vi "deleteController_TCrane.vi"() -> ()   [LabVIEW 2009]
uses:
  <vilib>/Platform/TimedLoop/XDataNode/nitl_modes.ctl
  <vilib>/Utility/miscctls.llb/LVRGBAColorTypeDef.ctl
  Instance           2 23Saved   OpenLoop_TCrane .vi
  <vilib>/Instr/_visa.llb/VISA Configure Serial Port (Instr).vi
  <vilib>/Platform/TimedLoop/XDataNode/XDataNode.xnode
  <vilib>/Platform/TimedLoop/XDataNode/loadlvalarms.vi
  <vilib>/Platform/TimedLoop/XDataNode/timing_clust.ctl
  <vilib>/Platform/TimedLoop/XDataNode/wakeup.ctl
  Instance           3 23Saved   OpenLoop_TCrane .vi
  Instance           4 23Saved   OpenLoop_TCrane .vi
  Instance           5 23Saved   OpenLoop_TCrane .vi
  <vilib>/Utility/file.llb/Read From Spreadsheet File (string).vi
  <vilib>/Utility/file.llb/Write To Spreadsheet File (DBL).vi
  <vilib>/Utility/file.llb/Write To Spreadsheet File (string).vi
  <vilib>/Utility/miscctls.llb/LV3DPointTypeDef.ctl
  <vilib>/imath/engines/lvmath2/RunTimeEngine/ErrorHandling/NIMS_Finalize Error.vi
  <vilib>/imath/engines/lvmath2/RunTimeEngine/Parser/MC_Version.vi
  <vilib>/imath/engines/lvmath2/RunTimeEngine/NodeEndStatement/NIMS_NodeEndStatement_Output.vi
  <instcachedir>/1/NIMS_NodeEndStatement_Output_53EC0D466D134D7ABD903AC30B43404B.lvgen/NIMS_NodeEndStatement_Output_53EC0D466D134D7ABD903AC30B43404B_004.vi
  <vilib>/imath/engines/lvmath2/RunTimeEngine/BuiltInFunctions/abs/NIMS_abs(signed).vi
  <instcachedir>/1/NIMS_abs(signed)_C4FCB8E6058B49B797C7C8D53CA5F6EC.lvgen/NIMS_abs(signed)_C4FCB8E6058B49B797C7C8D53CA5F6EC_000.vi
  <vilib>/imath/engines/lvmath/Functions/Error Handling/MergeErrorsWrapper.vi
  <instcachedir>/1/NIMS_NodeEndStatement_Output_53EC0D466D134D7ABD903AC30B43404B.lvgen/NIMS_NodeEndStatement_Output_53EC0D466D134D7ABD903AC30B43404B_002.vi
  RTDACUSB_TCrane.dll
  <vilib>/Platform/TimedLoop/XDataNode/XDNodeRunTimeDep.lvlib
panel:
  in  "Tab Control":enum32{"Main", "I/O", "Advanced", "Wireless"}(tab)
  in  "Motors on":bool caption="Motors"
  in  "Camera Control 2":dbl(slide)=60.0 min=1.0 max=90.0 scale=90.0..1.0
  out "X displacement chart":dbl(graph)
  out "Y displacement chart":dbl(graph)
  out "Z displacement chart":dbl(graph)
  out "XY Graph":cluster{"Y":dbl[], "Y":dbl[]}[](graph)
  out "Alpha":dbl
  out "Beta":dbl
  out "3D view":refnum<vi>(3d-picture)
  in  "Camera Control":dbl(slide) scale=-180.0..180.0
  in  "Animation":bool
  in  "Controller:":u16(ring) items=["None", "P (Tracking)", "P (Delay Controller)", "PI (Tracking)", "PID (DelayController)"]
  in  "X":dbl
  in  "Stop Controller":bool
  in  "T":dbl min=0.0 max=3.14 step=0.05
  in  "Z":dbl
  in  "Referense Slide X":dbl(slide) scale=0.0..50.0
  in  "Referense Slide T":dbl(slide) scale=0.0..3.14
  in  "Referense Slide Z":dbl(slide) scale=0.0..100.0
  in  "Cont Switch X":bool
  in  "Cont Switch T":bool
  in  "Cont Switch Z":bool
  in  "stop 2":bool
  in  "Home":bool
  in  "Reset angles":bool
  in  "Motors off":bool
  in  "Timed Sequence":bool
  in  "Stop TIV":bool
  in  "Saving":bool
  in  "Stop saving":bool
  in  "Start saving":bool
  in  "Path":path
  in  "Load TIV 2":path
  out "TIV Table":string[][](table)
  in  "Load TIV":bool
  out "TIV active":bool
  in  "Run TIV+SAVE":bool
  in  "Input type":bool
  out "Control Sequence":bool
  out "Reference Series\n(Trajectory)":bool
  out "Switch at":dbl
  out "X Scope":dynamicdata(graph)
  out "Theta Scope":dynamicdata(graph)
  out "Z Scope":dynamicdata(graph)
  out "Waveform Chart":i32(graph)
  out "Sample time [ms]":dbl format="%#.12g"
  out "Counter pulses":dbl format="%#.12g"
  out "Time":dbl
  in  "Timer active":bool
  out "Encoder X":dbl format="%#.12g"
  in  "X-axis control":dbl(slide) scale=-1.0..1.0
  in  "X-Motor On/Off":bool
  out "X - Motor On/Off":bool
  out "Numeric":dbl
  out "No of detected boards":dbl
  out "Logic version":dbl
  out "Last error":string
  in  "Theta-angle control":dbl(slide) scale=-1.0..1.0
  in  "T-Motor On/Off":bool
  out "Theta - Motor On/Off":bool
  out "Numeric 2":dbl
  in  "Z-axis control":dbl(slide) scale=-1.0..1.0
  in  "Z-Motor On/Off":bool
  out "Z - Motor On/Off":bool
  out "Numeric 3":dbl
  out "Encoder Theta":dbl format="%#.12g"
  out "Encoder Z":dbl format="%#.12g"
  out "Encoder Alfa":dbl format="%#.12g"
  out "Encoder Beta":dbl format="%#.12g"
  in  "Limit flags":T1(radio)=enum."Radio Selection 2"
  in  "Therm flags":T2(radio)=enum."Radio Selection 2"
  in  "Stop motors":bool
  out "X-axis therm flag":bool
  out "T-angle therm flag":bool
  out "Z-axis therm flag":bool
  out "X-axis limit flag":bool
  out "T-angle limit flag":bool
  out "Z-axis limit flag":bool
  in  "Reset encoders":bool
  out "RESET value":dbl format="%#.12g"
  in  "Soft limit flags":bool=TRUE
  in  "k 1":dbl=0.4 step=0.1
  in  "k 2":dbl=0.4 step=0.1
  in  "Mode":T3=enum."Discard missed periods, maintain original phase"
  in  "Wireless Active":bool
  in  "Baud Rate":i32(ring)=6 items=["2400"=2400, "4800"=4800, "9600"=9600, "19200"=19200, "38400"=38400, "57600"=57600, "115200"=115200]
  in  "VISA resource name":refnum<visa-resource-name>="COM1"
  out "Float1":sgl
  out "Float2":sgl
  out "Float3":sgl
  out "Float4":sgl
  out "Current Ref Z":dbl
  out "Current Ref X":dbl
  out "Current Ref T":dbl
  in  "Offset Beta":dbl
  in  "Offset Alpha":dbl
  out "TIV size":i32
  out "Index":i32
  # "Time"
  # "X"
  # "Theta"
  # "Z"
  # "Please specify the Input type when loading the input data chart"
  # "RT-DAC/USB status"
  # "Tower Crane motor control"
  # "Controller Parameters"
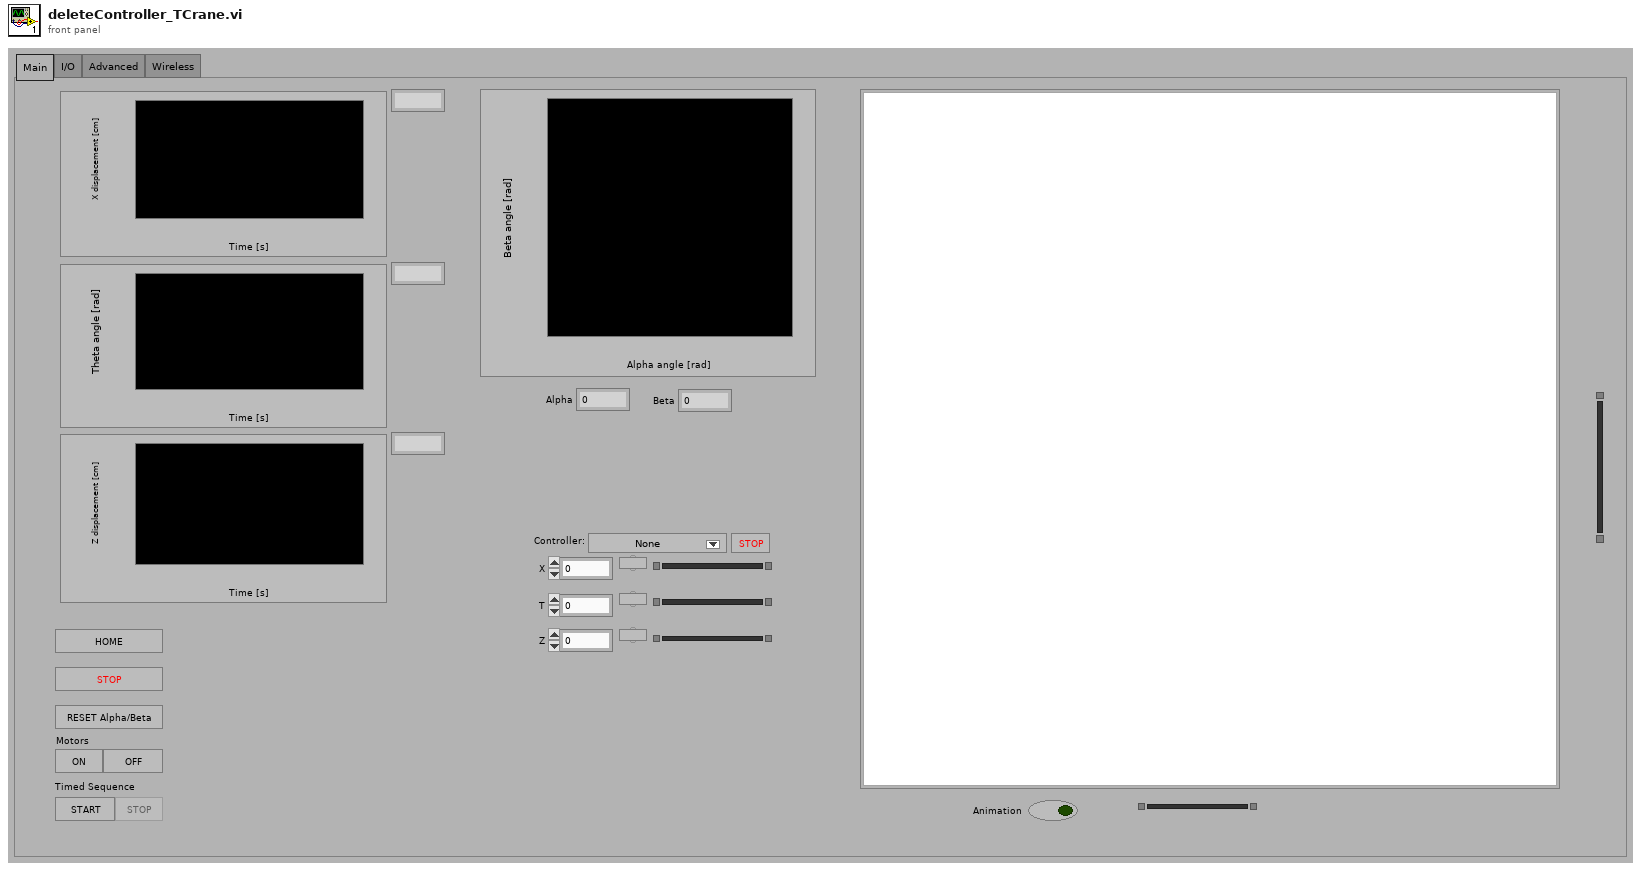
[diagram p1: front panel]
types:
  T1 = enum32{"Set limit flags to:", "Radio Selection 2"}
  T2 = enum32{"Set therm flags to:", "Radio Selection 2"}
  T3 = typedef "XDNodeRunTimeDep.lvlib/nitl_modes.ctl" = enum32{"No Change", "Process missed periods, maintain original phase", "Discard missed periods, maintain original phase", "Process missed periods, ignore original phase", "Discard missed periods, ignore original phase"}
  T4 = typedef "LVRGBAColorTypeDef.ctl" = cluster{"Red":sgl, "Green":sgl, "Blue":sgl, "Alpha":sgl}
  T5 = typedef "XDNodeRunTimeDep.lvlib/timing_clust.ctl" = cluster{"Expected End [f-1]":u64, "Actual End [f-1]":u64, "Finished Late? [f-1]":bool, "Expected End [i-1]":u64, "Actual End [i-1]":u64, "Finished Late? [i-1]":bool, "Expected Start [i]":u64, "Actual Start [i]":u64, "Expected Start [f]":u64, "Actual Start [f]":u64, "Source Name":string, "Structure Name":string, "Period":i64, "Deadline":i64, "Offset":i64, "Start":i64, "Priority":i32, "Timeout":i32, "Mode":T3, "Wakeup Reason":T6, "Error":errorcluster, "Source Type":string, "Secondary Source Type":string, "Global End Time":u64, "Global Start Time":u64, "Frame Duration":u64, "Iteration Duration":u64, "Assigned CPU":i32, "I/O Scan Engine Mode":u32}
  T6 = typedef "XDNodeRunTimeDep.lvlib/wakeup.ctl" = enum32{"Normal", "Aborted", "Asynchronous wakeup", "Timing source error", "Timed loop error", "Timeout"}
  T7 = typedef "LV3DPointTypeDef.ctl" = cluster{"X":sgl, "Y":sgl, "Z":sgl}
  T8 = enum8{"Enabled", "Disabled", "Disabled and Grayed Out"}
  T9 = cluster{"Numeric 2":dbl, "Numeric 3":dbl, "Numeric 4":dbl}
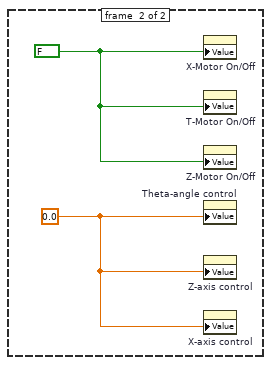
[diagram p2: hidden frame]
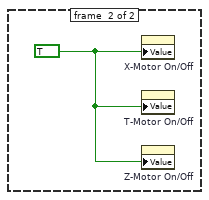
[diagram p3: hidden frame]
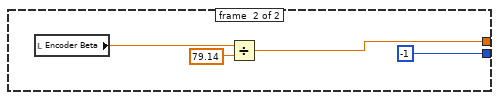
[diagram p4: hidden frame]
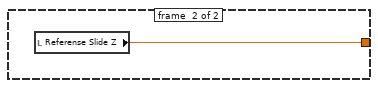
[diagram p5: hidden frame]
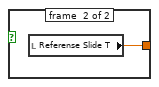
[diagram p6: hidden frame]
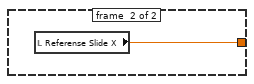
[diagram p7: hidden frame]
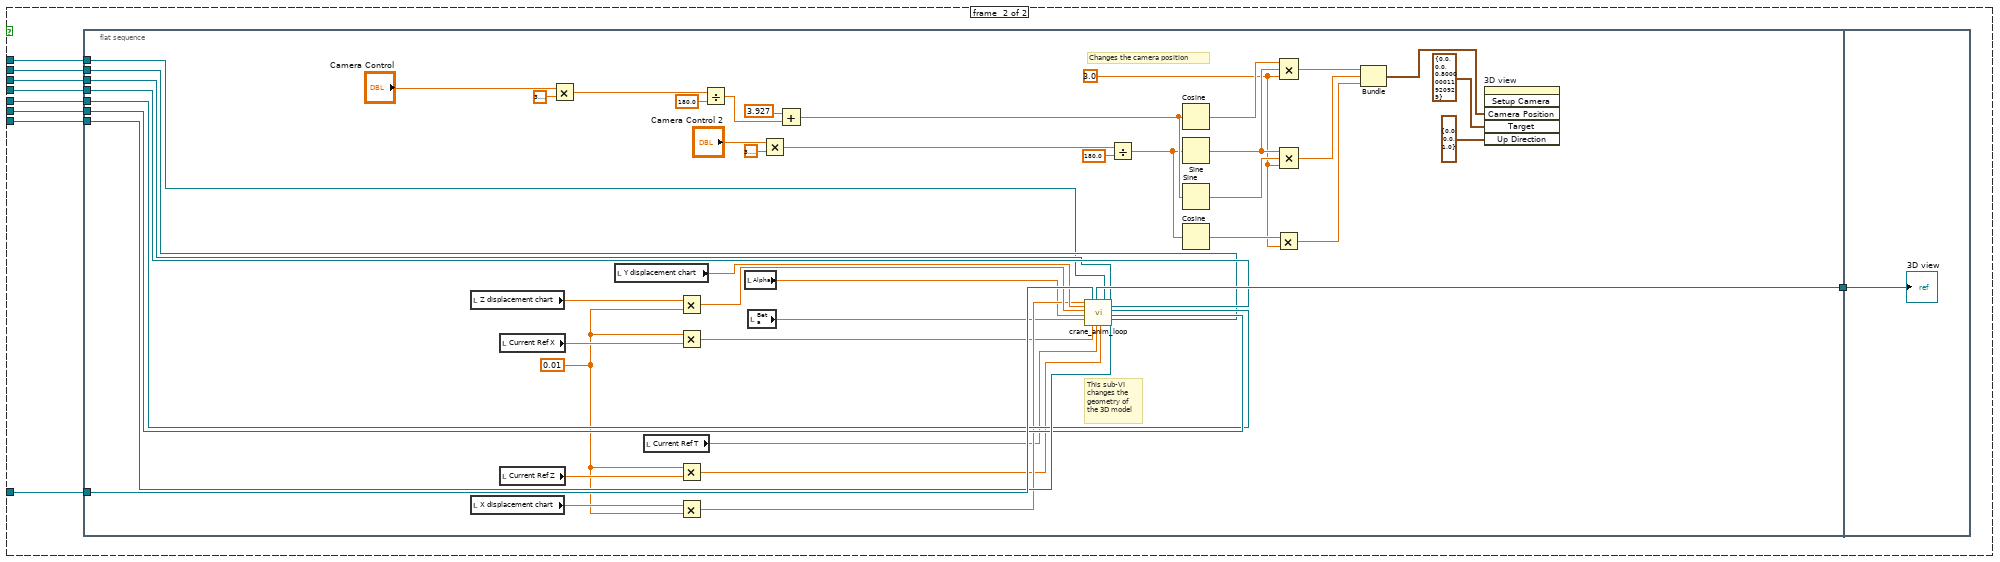
[diagram p8: hidden frame]
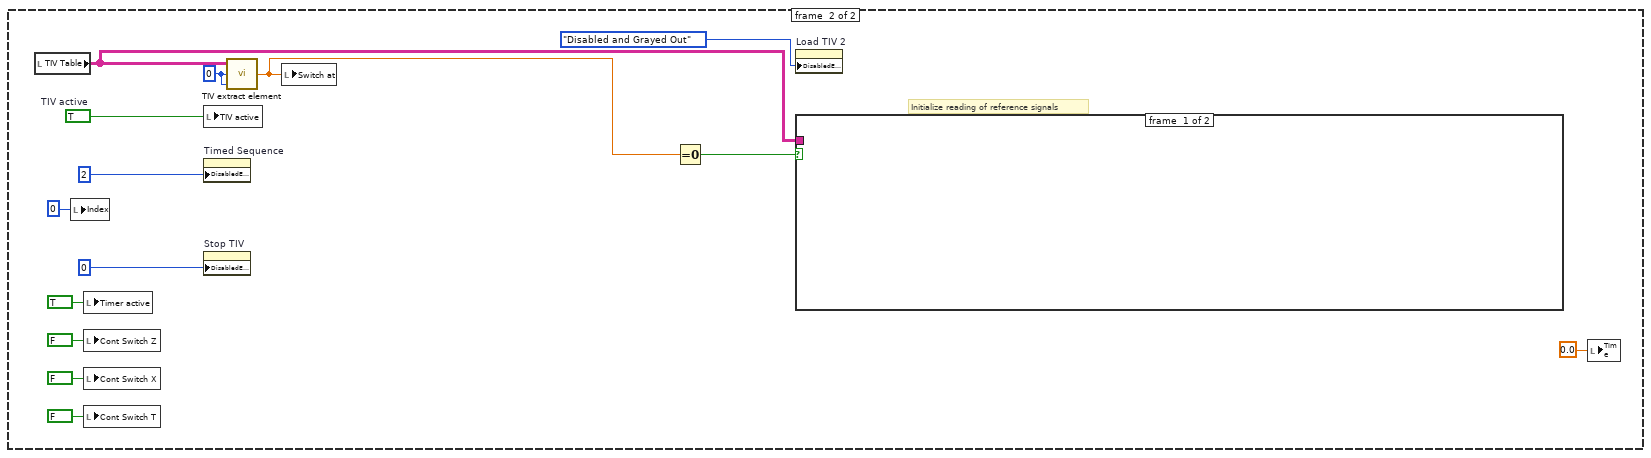
[diagram p9: hidden frame]
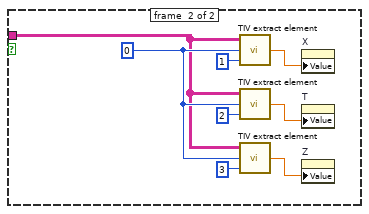
[diagram p10: hidden frame]
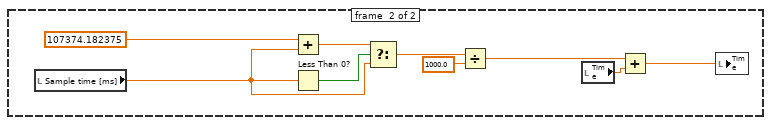
[diagram p11: hidden frame]
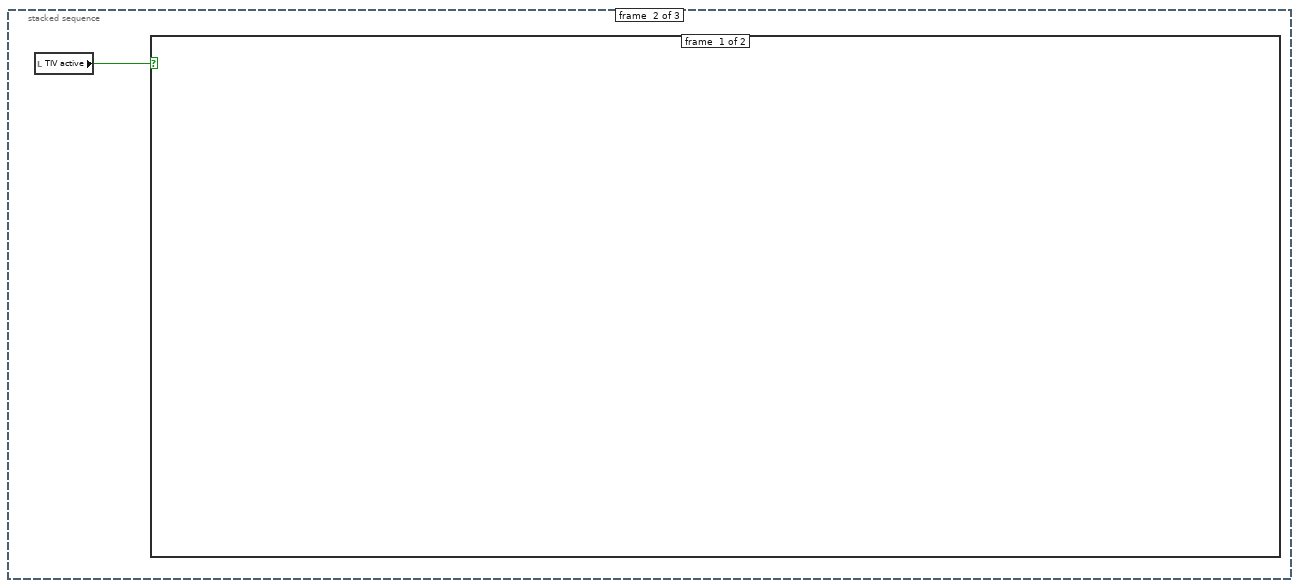
[diagram p12: hidden frame]
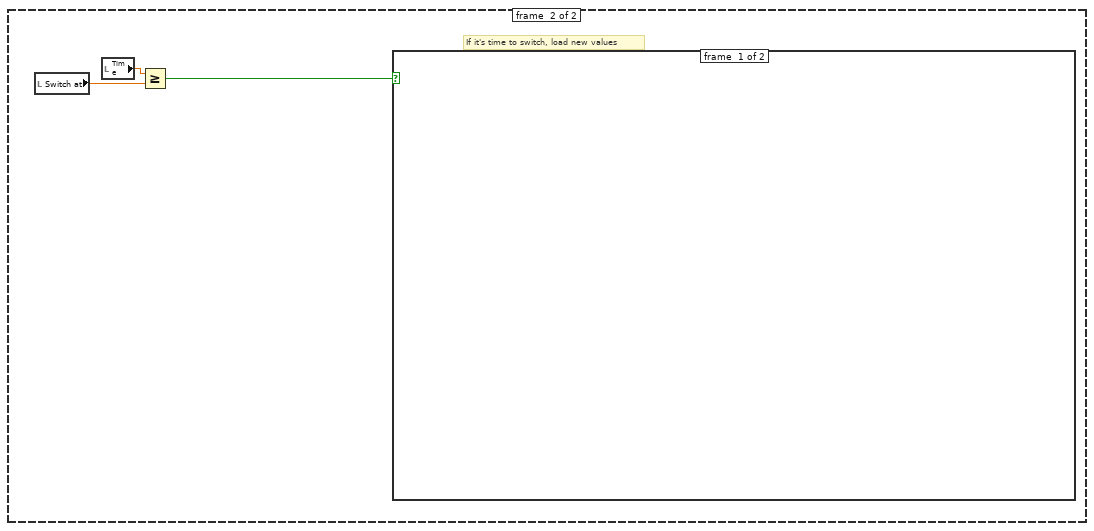
[diagram p13: hidden frame]
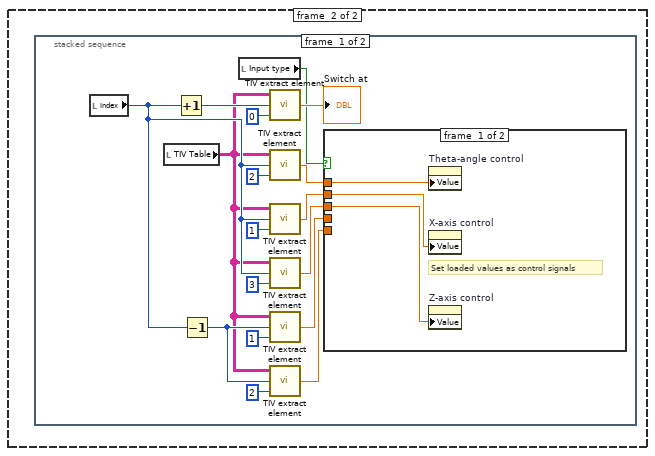
[diagram p14: hidden frame]
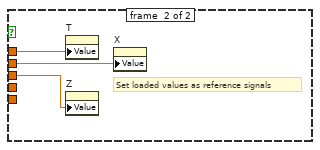
[diagram p15: hidden frame]
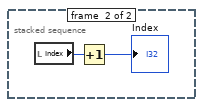
[diagram p16: hidden frame]
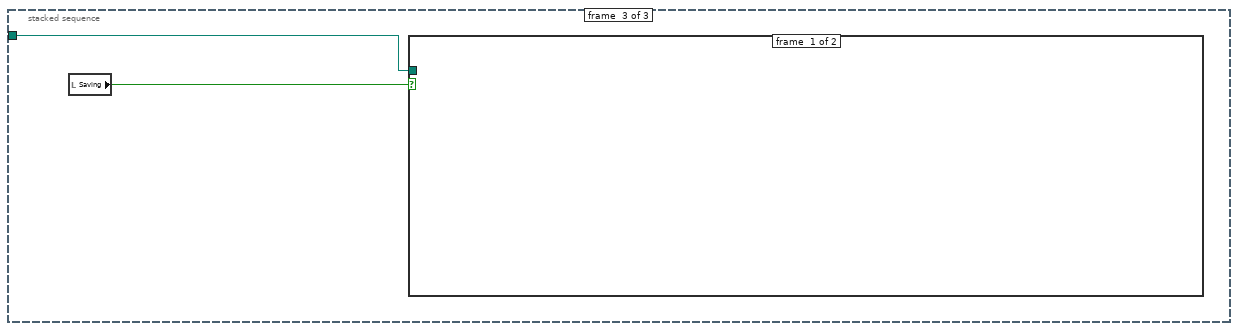
[diagram p17: hidden frame]
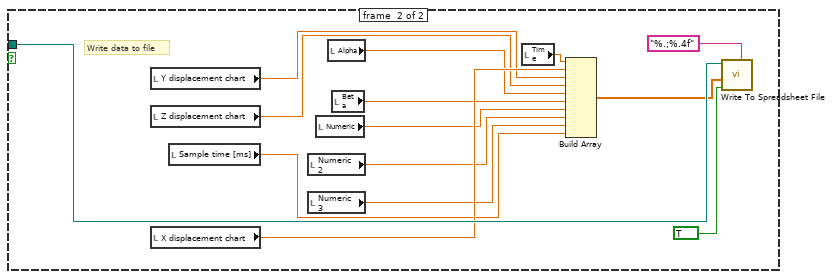
[diagram p18: hidden frame]
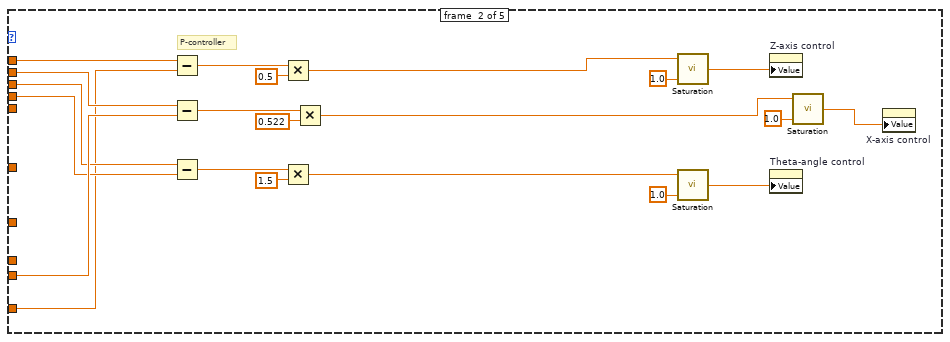
[diagram p19: hidden frame]
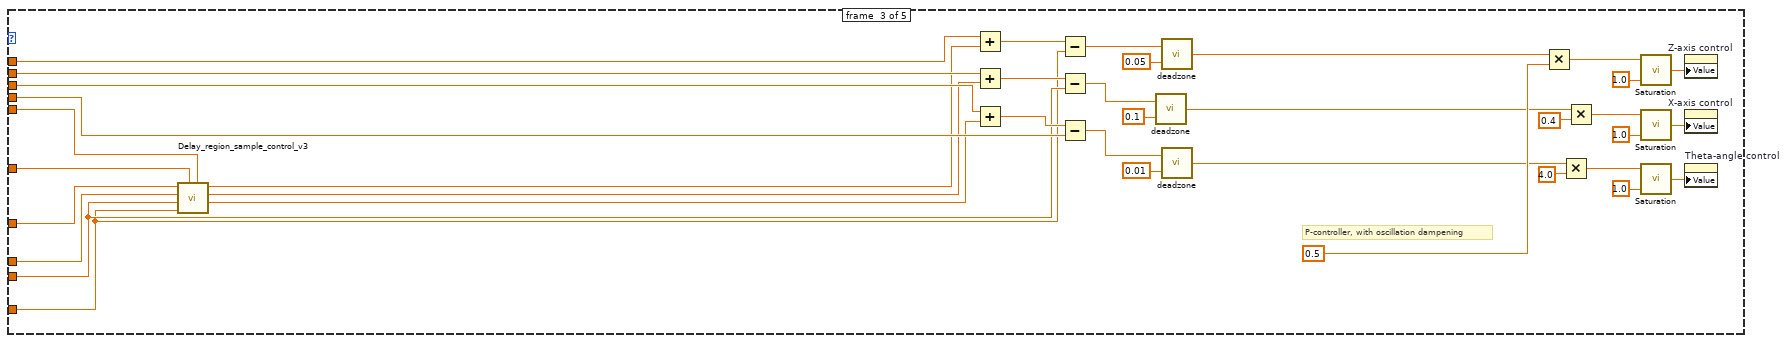
[diagram p20: hidden frame]
diagram:
  # "Close session to port."
  # "Read from the wireless connection"
  # "Initialize the file path controls"
  # "Initialization of the 3D animation.\nContained in a sub-VI to reduce clutter."
  n1 = call <vilib>:"Application Directory.vi"() -> ("Application Directory"=w16:path)
  n2 = property on="3D view" class="SceneGraphDisp (strict)"("Background Color"=T4 {"Red"=0.5, "Green"=0.5, "Blue"=0.5, "Alpha"=1.0}) -> ()  [unwired: 2 in, 2 out]
  n3 = Build Path(base path=w16, name or relative path="Outputs") -> (appended path=w18:path)
  n4 = dll-call lib="C:/Documents and Settings/student/Desktop/crane controller/RTDACUSB_TCrane.dll" fn="RTDACUSB_NoOfDetectedBoards" ("PlxApi.dll:PlxBusIopWrite")() -> ("pNoOfDetectedBoards"=w34:i32)  [unwired: 5 in, 2 out]
  "No of detected boards" <- w34
  n5 = Build Path(base path=w16, name or relative path="Inputs") -> (appended path=w17:path)
  n6 = local write "Load TIV 2"(w17) -> ()
  n7 = call "crane_anim_init.vi"() -> ("Trolley"=w22:refnum<vi>, "Main"=w29:refnum<vi>, "Pivot Beta"=w23:refnum<vi>, "Arm"=w24:refnum<vi>, "Load"=w25:refnum<vi>, "Target"=w28:refnum<vi>, "Load Line"=w26:refnum<vi>, "Pivot Alpha"=w27:refnum<vi>)  [unwired: 3 in]
  n8 = local write "Path"(w18) -> ()
  n9 = Less?(x=w34, y=1) -> (x < y?=w33:bool)
  n10 = call-poly "VISA Configure Serial Port"("VISA resource name"="VISA resource name", "timeout (10sec)"=u32 10000, "baud rate (9600)"="Baud Rate") -> ("VISA resource name out"=w12:refnum<visa-resource-name>, "error out"=w10:errorcluster)  [unwired: 7 in, 4 out]
  n11 = call "Display Message to User"("Enable"=w33) -> ("OK"=w31:bool)  [unwired: 9 in, 1 out]
  n12 = VISA Flush I/O Buffer(VISA resource name=w12, error in (no error)=w10) -> (VISA resource name out=w9:refnum<visa-resource-name>, error out=w11:errorcluster)  [unwired: 1 in]
  n13 = VISA Set I/O Buffer Size(VISA resource name=w9, size (4096)=u32 15 ("baud rate (9600)"), error in (no error)=w11) -> (VISA resource name out=w5:refnum<visa-resource-name>, error out=w6:errorcluster)  [unwired: 1 in]
  n14 = node-c288("Mode") -> (w21:T5)  [unwired: 9 in]
  n15 = timed-loop {
    tunnel: w31 -> [w242]
    tunnel: w29 -> [w241]
    tunnel: w28 -> [w240]
    tunnel: w27 -> [w239]
    tunnel: w26 -> [w238]
    tunnel: w25 -> [w237]
    tunnel: w24 -> [w236]
    tunnel: w23 -> [w235]
    tunnel: w22 -> [w234]
    timing: w21 -> [_]
    timing-out: [_] -> w20
    shift-right: [w41] -> w3
    shift-left: w5 -> [w40]
    shift-right: [w39] -> w2
    shift-left: w6 -> [w43]
    stop <- w44 stop-if-true
    w65 = 0.00153
    w177 = 0.00153
    w219 = 1
    w224 = 0
    # "Stops execution of"
    # "Stop saving of data"
    # "Turn off all the motors"
    # "Turn on all the motors"
    # "Initialize saving of data"
    # "Load the table from which the TIVs are read"
    # "Get reference signals"
    # "Take crane to home position"
    # "Stop the controller"
    # "Feed control signals, reference signals and measurements into the scopes"
    # "Animation update"
    # "When wireless reading is active\nthis value gets fed into the chart"
    n16 = node-c288() -> ()  [unwired: 1 in, 1 out]
    n17 = local read "Wireless Active"() -> (w42:bool)
    n18 = local read "TIV size"() -> (w144:i32)
    n19 = dll-call lib="C:/Documents and Settings/student/Desktop/crane controller/RTDACUSB_TCrane.dll" fn="RTDACUSB_LastError" ("PlxApi.dll:PlxBusIopWrite")() -> ("dsrp"=→"Last error":string)  [unwired: 3 in, 2 out]
    n20 = local read "Stop Controller"() -> (w123:bool)
    n21 = local read "Stop Controller"() -> (w126:bool)
    n22 = local read "Stop Controller"() -> (w129:bool)
    n23 = local read "Stop Controller"() -> (w46:bool)
    n24 = local read "Encoder Beta"() -> (w178:dbl)
    n25 = local read "Stop motors"() -> (w125:bool)
    n26 = local read "Stop motors"() -> (w128:bool)
    n27 = local read "Encoder Alfa"() -> (w179:dbl)
    n28 = local read "Stop motors"() -> (w45:bool)
    n29 = local read "Cont Switch Z"() -> (w77:bool)
    n30 = local read "Cont Switch X"() -> (w81:bool)
    n31 = local read "Cont Switch T"() -> (w79:bool)
    n32 = call "ReadFloats.vi"("VISA resource name in"=w40, "Enable"=w42, "error in"=w43) -> ("VISA resource name out"=w41:refnum<visa-resource-name>, "error out"=w39:errorcluster, "Float1"=→"Float1":sgl, "Float2"=→"Float2":sgl, "Float3"=→"Float3":sgl, "Float4"=→"Float4":sgl)  [unwired: 10 in, 1 out]
    n33 = case shown="True" "Load TIV" {
      frame #0 {
      }
      frame #1 {
        n34 = stacked-sequence {
          frame #0 {
            n35 = call-poly <vilib>:"Read From Spreadsheet File.vi"("file path (dialog if empty)"="Load TIV 2") -> ("all rows"=→"TIV Table":string[][])  [unwired: 6 in, 4 out]
          }
          frame #1 {
            n36 = local read "TIV Table"() -> (w945:string[][])
            n37 = Array Size(array=w945) -> (size(s)=w946:i32[])
            n38 = Index Array(array=w946, index=0) -> (element=→"TIV size":i32)
          }
        }
      }
    }
    n39 = case shown="True" "Motors on" {
      frame #0 {
      }
      frame #1 {
        w245 = TRUE ("X-Motor On/Off")
        n40 = property on="X-Motor On/Off" class="Bool (strict)"("Value"=w245) -> ()  [unwired: 2 in, 2 out]
        n41 = property on="T-Motor On/Off" class="Bool (strict)"("Value"=w245) -> ()  [unwired: 2 in, 2 out]
        n42 = property on="Z-Motor On/Off" class="Bool (strict)"("Value"=w245) -> ()  [unwired: 2 in, 2 out]
      }
    }
    n43 = local read "Index"() -> (w143:i32)
    n44 = case shown="True" "Animation" {
      tunnel: w241 -> [_ w267]
      tunnel: w240 -> [_ w266]
      tunnel: w239 -> [_ w265]
      tunnel: w238 -> [_ w264]
      tunnel: w237 -> [_ w263]
      tunnel: w236 -> [_ w262]
      tunnel: w235 -> [_ w261]
      tunnel: w234 -> [_ w260]
      frame #0 {
      }
      frame #1 {
        n45 = flat-sequence {
          tunnel: [w308] -> w268
          tunnel: w267 -> [w307]
          tunnel: w266 -> [w306]
          tunnel: w265 -> [w305]
          tunnel: w264 -> [w304]
          tunnel: w263 -> [w303]
          tunnel: w262 -> [w302]
          tunnel: w261 -> [w301]
          tunnel: w260 -> [w300]
          tunnel: w268 -> [w314]
          frame #0 {
            w269 = 3.0 ("y")
            w285 = 0.01 ("y")
            # "Changes the camera position"
            # "This sub-VI\nchanges the\ngeometry of\nthe 3D model"
            n46 = local read "Z displacement chart"() -> (w293:dbl)
            n47 = local read "X displacement chart"() -> (w290:dbl)
            n48 = local read "Current Ref X"() -> (w286:dbl)
            n49 = local read "Current Ref Z"() -> (w287:dbl)
            n50 = Multiply(x="Camera Control", y=3.141592653589793) -> (x*y=w295:dbl)
            n51 = local read "Y displacement chart"() -> (w299:dbl)
            n52 = local read "Current Ref T"() -> (w284:dbl)
            n53 = Multiply(x=w293, y=w285) -> (x*y=w292:dbl)
            n54 = Multiply(x=w285, y=w286) -> (x*y=w289:dbl)
            n55 = Multiply(x=w285, y=w287) -> (x*y=w288:dbl)
            n56 = Multiply(x=w290, y=w285) -> (x*y=w291:dbl)
            n57 = Divide(x=w295, y=180.0) -> (x/y=w296:dbl)
            n58 = local read "Alpha"() -> (w276:dbl)
            n59 = local read "Beta"() -> (w275:dbl)
            n60 = Multiply(x="Camera Control 2", y=3.141592653589793) -> (x*y=w282:dbl)
            n61 = Add(x=3.927, y=w296) -> (x+y=w312:dbl)
            n62 = call "crane_anim_loop.vi"("X"=w291, "Theta"=w299, "Z"=w292, "Alpha"=w276, "Beta"=w275, "Main in"=w307, "Target X"=w289, "Target Theta"=w284, "Target Z"=w288, "Trolley"=w300, "Arm"=w302, "Load"=w303, "Load Line"=w304, "Pivot Alpha"=w305, "Pivot Beta"=w301, "Target"=w306) -> ("Main out"=w308:refnum<vi>)  [unwired: 3 in]
            n63 = Divide(x=w282, y=180.0) -> (x/y=w279:dbl)
            n64 = Cosine(x=w312) -> (cos(x)=w274:dbl)
            n65 = Sine(x=w279) -> (sin(x)=w271:dbl)
            n66 = Sine(x=w312) -> (sin(x)=w270:dbl)
            n67 = Cosine(x=w279) -> (cos(x)=w277:dbl)
            n68 = Multiply(x=w277, y=w269) -> (x*y=w278:dbl)
            n69 = Compound Arithmetic op=MULTIPLY(w274, w271, w269) -> (w273:dbl)
            n70 = Compound Arithmetic op=MULTIPLY(w271, w270, w269) -> (w272:dbl)
            n71 = Bundle(w273, w272, w278) -> (w309:cluster{dbl, dbl, dbl})  [unwired: 1 in]
            n72 = invoke on="3D view" class="SceneGraphDisp (strict)" method="Setup Camera"("Camera Position"=w309, "Target"=T7 {"X"=0.0, "Y"=0.0, "Z"=0.8}, "Up Direction"=T7 {"X"=0.0, "Y"=0.0, "Z"=1.0}) -> ()  [unwired: 3 in, 6 out]
          }
          frame #1 {
            "3D view" <- w314
          }
        }
      }
    }
    n73 = case shown="True" "Home" {
      frame #0 {
      }
      frame #1 {
        n74 = local read "T-angle limit flag"() -> (w950:bool)
        n75 = local read "Z-axis limit flag"() -> (w949:bool)
        n76 = local read "X-axis limit flag"() -> (w951:bool)
        n77 = Not(x=w949) -> (.not. x?=w954:bool)
        n78 = Not(x=w950) -> (.not. x?=w958:bool)
        n79 = Not(x=w951) -> (.not. x?=w961:bool)
        n80 = Compound Arithmetic op=AND(w949, w950, w951) -> (invert w948:bool)
        n81 = Boolean To (0,1)(Boolean=w954) -> (0, 1=w955:i16)
        n82 = property on="Home" class="Bool (strict)"("Value"=w948) -> ()  [unwired: 2 in, 2 out]
        n83 = Boolean To (0,1)(Boolean=w958) -> (0, 1=w959:i16)
        n84 = Boolean To (0,1)(Boolean=w961) -> (0, 1=w963:i16)
        n85 = Multiply(x=w955, y=-1) -> (x*y=w952:i32)
        n86 = Multiply(x=w959, y=-1) -> (x*y=w956:i32)
        n87 = Multiply(x=w963, y=-1) -> (x*y=w962:i32)
        n88 = property on="Z-axis control" class="Slide (strict)"("Value"=w952) -> ()  [unwired: 2 in, 2 out]
        n89 = property on="Theta-angle control" class="Slide (strict)"("Value"=w956) -> ()  [unwired: 2 in, 2 out]
        n90 = property on="X-axis control" class="Slide (strict)"("Value"=w962) -> ()  [unwired: 2 in, 2 out]
      }
    }
    n91 = Or(x=w242, y="stop 2") -> (x .or. y?=w44:bool)
    n92 = Equal?(x=w143, y=w144) -> (x = y?=w145:bool)
    n93 = local read "T-angle limit flag"() -> (w169:bool)
    n94 = local read "X-axis limit flag"() -> (w159:bool)
    n95 = local read "Z-axis limit flag"() -> (w75:bool)
    n96 = local read "Soft limit flags"() -> (w141:bool)
    n97 = local read "Soft limit flags"() -> (w140:bool)
    n98 = case shown="False" w79 {
      tunnel: [w256 w257] -> w78
      frame #0 {
        n99 = local read "T"() -> (w256:dbl)
      }
      frame #1 {
        n100 = local read "Referense Slide T"() -> (w257:dbl)
      }
    }
    n101 = local read "Theta-angle control"() -> (w88:dbl)
    n102 = Multiply(x=w179, y=w177) -> (x*y=w181:dbl)
    n103 = Multiply(x=w178, y=w177) -> (x*y=w180:dbl)
    n104 = case shown="False" w77 {
      tunnel: [w254 w255] -> w76
      frame #0 {
        n105 = local read "Z"() -> (w254:dbl)
      }
      frame #1 {
        n106 = local read "Referense Slide Z"() -> (w255:dbl)
      }
    }
    n107 = case shown="True" "Stop Controller" {
      frame #0 {
      }
      frame #1 {
        w913 = u16 0 items=["None", "P"] ("Controller:")
        n108 = property on="Controller:" class="Ring (strict)"("Value"=w913) -> ()  [unwired: 2 in, 2 out]
      }
    }
    n109 = case shown="False" w81 {
      tunnel: [w258 w259] -> w80
      frame #0 {
        n110 = local read "X"() -> (w258:dbl)
      }
      frame #1 {
        n111 = local read "Referense Slide X"() -> (w259:dbl)
      }
    }
    n112 = Stop(stop? (T)=w44) -> ()
    n113 = Or(x=w123, y=w125) -> (x .or. y?=w124:bool)
    n114 = Or(x=w126, y=w128) -> (x .or. y?=w127:bool)
    n115 = Or(x=w129, y="Stop motors") -> (x .or. y?=w130:bool)
    n116 = Or(x="Timed Sequence", y="Run TIV+SAVE") -> (x .or. y?=w108:bool)
    n117 = Or(x="Run TIV+SAVE", y="Timed Sequence") -> (x .or. y?=w105:bool)
    n118 = Or(x="Run TIV+SAVE", y="Start saving") -> (x .or. y?=w134:bool)
    n119 = Not(x="Input type") -> (.not. x?=→"Control Sequence":bool)
    n120 = Not(x="Input type") -> (.not. x?=w106:bool)
    n121 = local read "Y displacement chart"() -> (w119:dbl)
    n122 = local read "X displacement chart"() -> (w121:dbl)
    n123 = local read "Z displacement chart"() -> (w122:dbl)
    n124 = local read "Y displacement chart"() -> (w95:dbl)
    n125 = local read "Limit flags"() -> (w160:T1)
    n126 = local read "Limit flags"() -> (w172:T1)
    n127 = local read "Limit flags"() -> (w163:T1)
    n128 = Select(t="Referense Slide Z", s="Cont Switch Z", f="Z") -> (s? t:f=w61:dbl)
    "Current Ref Z" <- w61
    n129 = Select(t="Referense Slide X", s="Cont Switch X", f="X") -> (s? t:f=w62:dbl)
    "Current Ref X" <- w62
    n130 = Select(t="Referense Slide T", s="Cont Switch T", f="T") -> (s? t:f=w115:dbl)
    "Current Ref T" <- w115
    n131 = dll-call lib="C:/Documents and Settings/student/Desktop/crane controller/RTDACUSB_TCrane.dll" fn="RTDACUSB_Receive" ("PlxApi.dll:PlxBusIopWrite")("pLogicVersion"=w224, "pApplicationName"="TestInTeCo", "pCN1Direction"=w224, "pCN1Input"=w224, "pPWMDivider"=w224, "pPWMWidth0"=w224, "pPWMWidth1"=w224, "pPWMWidth2"=w224, "pPWMDir0"=w224, "pPWMDir1"=w224, "pPWMDir2"=w224, "pPWMBrake0"=w224, "pPWMBrake1"=w224, "pPWMBrake2"=w224, "pPWMTherm0"=w224, "pPWMTherm1"=w224, "pPWMTherm2"=w224, "pPWMThermFlag0"=w224, "pPWMThermFlag1"=w224, "pPWMThermFlag2"=w224, "pNOFlag"=w224, "pLimitActive0"=w224, "pLimitActive1"=w224, "pLimitActive2"=w224, "pLimitFlag0"=w224, "pLimitFlag1"=w224, "pLimitFlag2"=w224, "pLimit0"=w224, "pLimit1"=w224, "pLimit2"=w224, "pEncoderReset0"=w224, "pEncoderReset1"=w224, "pEncoderReset2"=w224, "pEncoderReset3"=w224, "pEncoderReset4"=w224, "pEncoderAutoResetFlag0"=w224, "pEncoderAutoResetFlag1"=w224, "pEncoderAutoResetFlag2"=w224, "pEncoder0"=w224, "pEncoder1"=w224, "pEncoder2"=w224, "pEncoder3"=w224, "pEncoder4"=w224, "pTmrCnt0_Reset"=w224, "pTmrCnt0_Mode"=w224, "pTmrCnt0_Counter"=w224) -> ("pLogicVersion"=→"Logic version":u32, "pPWMThermFlag0"=w200:u32, "pPWMThermFlag1"=w201:u32, "pPWMThermFlag2"=w202:u32, "pLimitActive0"=w176:u32, "pLimitActive1"=w174:u32, "pLimitActive2"=w175:u32, "pEncoder0"=w57:i32, "pEncoder1"=w186:i32, "pEncoder2"=w182:i32, "pEncoder3"=w136:i32, "pEncoder4"=w135:i32, "pTmrCnt0_Counter"=w225:u32)  [unwired: 37 in, 2 out]
    "Counter pulses" <- w225
    "Encoder Theta" <- w186
    "Encoder Z" <- w182
    n132 = Or(x="Stop saving", y=w44) -> (x .or. y?=w151:bool)
    n133 = And(x=w108, y=w106) -> (x .and. y?=w107:bool)
    n134 = And(x=w105, y="Input type") -> (x .and. y?=w104:bool)
    n135 = Compound Arithmetic op=OR(w46, "Motors off", w45) -> (w48:bool)
    n136 = feedback #1() -> (w74:dbl)  [unwired: 1 in]
    n137 = feedback #2() -> (w70:dbl)  [unwired: 1 in]
    n138 = Multiply(x=w88, y=5) -> (x*y=w86:dbl)
    n139 = Merge Signals(w95, w78, w86) -> (→"Theta Scope":dynamicdata)
    n140 = local read "TIV active"() -> (w109:bool)
    n141 = Or(x=w145, y="Stop TIV") -> (x .or. y?=w110:bool)
    n142 = for {
      N: 10 -> [_]
      tunnel: w180 -> [w991]
      tunnel: w181 -> [w992]
      tunnel: [w992] -> w192 mode=indexing
      tunnel: [w991] -> w191 mode=indexing
    }
    n143 = case shown="True" w48 {
      frame #0 {
      }
      frame #1 {
        w243 = 0.0 ("Theta-angle control")
        w244 = FALSE ("T-Motor On/Off")
        n144 = property on="X-Motor On/Off" class="Bool (strict)"("Value"=w244) -> ()  [unwired: 2 in, 2 out]
        n145 = property on="T-Motor On/Off" class="Bool (strict)"("Value"=w244) -> ()  [unwired: 2 in, 2 out]
        n146 = property on="Z-Motor On/Off" class="Bool (strict)"("Value"=w244) -> ()  [unwired: 2 in, 2 out]
        n147 = property on="Theta-angle control" class="Slide (strict)"("Value"=w243) -> ()  [unwired: 2 in, 2 out]
        n148 = property on="Z-axis control" class="Slide (strict)"("Value"=w243) -> ()  [unwired: 2 in, 2 out]
        n149 = property on="X-axis control" class="Slide (strict)"("Value"=w243) -> ()  [unwired: 2 in, 2 out]
      }
    }
    n150 = case shown="True" w107 {
      frame #0 {
      }
      frame #1 {
        w922 = 0 ("Row")
        w924 = TRUE  # TIV active
        # "Initialize reading of control signals"
        n151 = local read "TIV Table"() -> (w919:string[][])
        n152 = local write "Index"(0 ("Index")) -> ()
        n153 = local write "Timer active"(TRUE ("Timer active")) -> ()
        n154 = local write "TIV active"(w924) -> ()
        n155 = property on="Load TIV" class="Bool"("DisabledEnum"=2) -> ()  [unwired: 2 in, 2 out]
        n156 = property on="Timed Sequence" class="Bool"("DisabledEnum"=2) -> ()  [unwired: 2 in, 2 out]
        n157 = property on="Stop TIV" class="Bool"("DisabledEnum"=0) -> ()  [unwired: 2 in, 2 out]
        n158 = call "TIV extract element.vi"("Column"=w922, "Row"=w922, "Table"=w919) -> ("Element"=w921:dbl)
        n159 = local write "Switch at"(w921) -> ()
        n160 = Equal To 0?(x=w921) -> (x = 0?=w920:bool)
        n161 = property on="Load TIV 2" class="Path"("DisabledEnum"=T8."Disabled and Grayed Out" ("Disabled")) -> ()  [unwired: 2 in, 2 out]
        n162 = case shown="True" w920 {
          tunnel: w919 -> [_ w935]
          frame #0 {
          }
          frame #1 {
            w934 = 0 ("Row")
            n163 = call "TIV extract element.vi"("Column"=1, "Row"=w934, "Table"=w935) -> ("Element"=w928:dbl)
            n164 = call "TIV extract element.vi"("Column"=2, "Row"=w934, "Table"=w935) -> ("Element"=w930:dbl)
            n165 = call "TIV extract element.vi"("Column"=3, "Row"=w934, "Table"=w935) -> ("Element"=w929:dbl)
            n166 = property on="X-axis control" class="Slide (strict)"("Value"=w928) -> ()  [unwired: 2 in, 2 out]
            n167 = property on="Theta-angle control" class="Slide (strict)"("Value"=w930) -> ()  [unwired: 2 in, 2 out]
            n168 = property on="Z-axis control" class="Slide (strict)"("Value"=w929) -> ()  [unwired: 2 in, 2 out]
          }
        }
        "Time" <- 0.0 ("Time")
      }
    }
    n169 = case shown="True" w104 {
      frame #0 {
      }
      frame #1 {
        w323 = 0 ("Column")
        w326 = TRUE  # TIV active
        # "Initialize reading of reference signals"
        n170 = local read "TIV Table"() -> (w319:string[][])
        n171 = local write "Index"(0 ("Index")) -> ()
        n172 = local write "Timer active"(TRUE ("Timer active")) -> ()
        n173 = local write "Cont Switch Z"(FALSE ("Cont Switch Z")) -> ()
        n174 = local write "Cont Switch X"(FALSE ("Cont Switch X")) -> ()
        n175 = local write "Cont Switch T"(FALSE ("Cont Switch T")) -> ()
        n176 = local write "TIV active"(w326) -> ()
        n177 = property on="Timed Sequence" class="Bool"("DisabledEnum"=2) -> ()  [unwired: 2 in, 2 out]
        n178 = property on="Stop TIV" class="Bool"("DisabledEnum"=0) -> ()  [unwired: 2 in, 2 out]
        n179 = call "TIV extract element.vi"("Column"=w323, "Row"=w323, "Table"=w319) -> ("Element"=w322:dbl)
        n180 = local write "Switch at"(w322) -> ()
        n181 = Equal To 0?(x=w322) -> (x = 0?=w320:bool)
        n182 = property on="Load TIV 2" class="Path"("DisabledEnum"=T8."Disabled and Grayed Out" ("Disabled")) -> ()  [unwired: 2 in, 2 out]
        n183 = case shown="True" w320 {
          tunnel: w319 -> [_ w332]
          frame #0 {
          }
          frame #1 {
            w336 = 0 ("Row")
            n184 = call "TIV extract element.vi"("Column"=1, "Row"=w336, "Table"=w332) -> ("Element"=w329:dbl)
            n185 = call "TIV extract element.vi"("Column"=2, "Row"=w336, "Table"=w332) -> ("Element"=w330:dbl)
            n186 = call "TIV extract element.vi"("Column"=3, "Row"=w336, "Table"=w332) -> ("Element"=w331:dbl)
            n187 = property on="X" class="DigNum (strict)"("Value"=w329) -> ()  [unwired: 2 in, 2 out]
            n188 = property on="T" class="DigNum (strict)"("Value"=w330) -> ()  [unwired: 2 in, 2 out]
            n189 = property on="Z" class="DigNum (strict)"("Value"=w331) -> ()  [unwired: 2 in, 2 out]
          }
        }
        n190 = local write "Time"(0.0 ("Time")) -> ()
      }
    }
    n191 = case shown="True" w134 {
      tunnel: "Path" -> [w973 w982]
      tunnel: [w973 w977] -> w49
      frame #0 {
      }
      frame #1 {
        n192 = local write "Time"(0.0 ("Time")) -> ()
        n193 = property on="Start saving" class="Bool"("DisabledEnum"=2) -> ()  [unwired: 2 in, 2 out]
        n194 = property on="Stop saving" class="Bool"("DisabledEnum"=0) -> ()  [unwired: 2 in, 2 out]
        n195 = Open/Create/Replace File(file path (use dialog)=w982, operation (0:open)=5, access (0:read/write)=2) -> (refnum out=w988:refnum<file>, cancelled=w981:bool, error out=w985:errorcluster)  [unwired: 3 in]
        n196 = Concatenate Strings("cdm = [", "\r\n") -> (w984:string)
        n197 = Not(x=w981) -> (.not. x?=w975:bool)
        n198 = local write "Saving"(w975) -> ()
        n199 = Write to Text File(file (use dialog)=w988, text=w984, error in=w985) -> (refnum out=w987:refnum<file>, error out=w986:errorcluster)  [unwired: 1 in, 1 out]
        n200 = local write "Timer active"(w975) -> ()
        n201 = Close File(refnum=w987, error in=w986) -> (path=w977:path, error out=w976:errorcluster)
        n202 = call <vilib>:"Simple Error Handler.vi"("error in (no error)"=w976) -> ()  [unwired: 4 in, 5 out]
      }
    }
    n203 = call "LimitFlagActionSoftLinearizedZ.vi"("Soft"="Soft limit flags", "Axis limit flag"=w75, "Old Control"=w74, "Global limit flag active"=w163, "Stop motors global"=w130, "Stop motor local"="Z-Motor On/Off", "Axis control signal"="Z-axis control") -> ("Slider control"=w73:dbl, "PWM Brake"=w68:u32, "PWM Direction"=w165:u32, "PWM width"=w164:u32)
    n204 = call "LimitFlagActionSoftLinearizedX.vi"("Soft"=w140, "Axis limit flag"=w159, "Old Control"=w70, "Global limit flag active"=w160, "Stop motors global"=w124, "Stop motor local"="X-Motor On/Off", "Axis control signal"="X-axis control") -> ("Slider control"=w69:dbl, "PWM Brake"=w156:u32, "PWM Direction"=w155:u32, "PWM width"=w154:u32)
    n205 = feedback #3() -> (w72:dbl)  [unwired: 1 in]
    n206 = call "LimitFlagActionSoftLinearizedT.vi"("Soft"=w141, "Axis limit flag"=w169, "Old Control"=w72, "Global limit flag active"=w172, "Stop motors global"=w127, "Stop motor local"="T-Motor On/Off", "Axis control signal"="Theta-angle control") -> ("Slider control"=w71:dbl, "PWM Brake"=w168:u32, "PWM Direction"=w167:u32, "PWM width"=w166:u32)
    n207 = Boolean To (0,1)(Boolean="Reset encoders") -> (0, 1=w189:i16)
    "RESET value" <- w189
    n208 = local read "Alpha"() -> (w53:dbl)
    n209 = local read "Beta"() -> (w52:dbl)
    n210 = case shown="3" "Controller:" {
      tunnel: w121 -> [_ w411 w425 w467 w653]
      tunnel: w62 -> [_ w412 w448 w468 w680]
      tunnel: w115 -> [_ w401 w447 w465 w679]
      tunnel: w119 -> [_ w400 w443 w466 w675]
      tunnel: w61 -> [_ w394 w449 w471 w681]
      tunnel: w122 -> [_ w393 w424 w469 w652]
      tunnel: "k 1" -> [_ _ w423 _ w651]
      tunnel: "k 2" -> [_ _ w432 _ w650]
      tunnel: w53 -> [_ _ w422 _ w655]
      tunnel: w52 -> [_ _ w421 _ w654]
      frame #0 {
        # "No controller"
      }
      frame #1 {
        # "P-controller"
        n211 = Subtract(x=w394, y=w393) -> (x-y=w398:dbl)
        n212 = Subtract(x=w412, y=w411) -> (x-y=w410:dbl)
        n213 = Subtract(x=w401, y=w400) -> (x-y=w405:dbl)
        n214 = Multiply(x=w398, y=0.5) -> (x*y=w396:dbl)
        n215 = Multiply(x=w405, y=1.5) -> (x*y=w403:dbl)
        n216 = Multiply(x=w410, y=0.522) -> (x*y=w407:dbl)
        n217 = call "Saturation.vi"("Limit"=1.0, "Input"=w396) -> ("Output"=w392:dbl)
        n218 = call "Saturation.vi"("Limit"=1.0, "Input"=w403) -> ("Output"=w399:dbl)
        n219 = property on="Z-axis control" class="Slide (strict)"("Value"=w392) -> ()  [unwired: 2 in, 2 out]
        n220 = property on="Theta-angle control" class="Slide (strict)"("Value"=w399) -> ()  [unwired: 2 in, 2 out]
        n221 = call "Saturation.vi"("Limit"=1.0, "Input"=w407) -> ("Output"=w408:dbl)
        n222 = property on="X-axis control" class="Slide (strict)"("Value"=w408) -> ()  [unwired: 2 in, 2 out]
      }
      frame #2 {
        # "P-controller, with oscillation dampening"
        n223 = call "Delay_region_sample_control_v3.vi"("K2"=w432, "K1"=w423, "Z"=w424, "X"=w425, "Beta"=w421, "Alpha"=w422) -> ("delta_T"=w426:dbl, "delta_X"=w427:dbl, "delta_Z"=w428:dbl)  [unwired: 1 in]
        n224 = Add(x=w449, y=w428) -> (x+y=w446:dbl)
        n225 = Add(x=w448, y=w427) -> (x+y=w445:dbl)
        n226 = Add(x=w447, y=w426) -> (x+y=w444:dbl)
        n227 = Subtract(x=w446, y=w424) -> (x-y=w416:dbl)
        n228 = Subtract(x=w445, y=w425) -> (x-y=w431:dbl)
        n229 = Subtract(x=w444, y=w443) -> (x-y=w419:dbl)
        n230 = call "deadzone.vi"("threshold"=0.1, "in"=w431) -> ("out"=w430:dbl)
        n231 = call "deadzone.vi"("threshold"=0.05, "in"=w416) -> ("out"=w417:dbl)
        n232 = call "deadzone.vi"("threshold"=0.01, "in"=w419) -> ("out"=w420:dbl)
        n233 = Multiply(x=w417, y=0.5) -> (x*y=w437:dbl)
        n234 = Multiply(x=w420, y=4.0) -> (x*y=w440:dbl)
        n235 = Multiply(x=w430, y=0.4) -> (x*y=w442:dbl)
        n236 = call "Saturation.vi"("Limit"=1.0, "Input"=w437) -> ("Output"=w434:dbl)
        n237 = call "Saturation.vi"("Limit"=1.0, "Input"=w442) -> ("Output"=w435:dbl)
        n238 = call "Saturation.vi"("Limit"=1.0, "Input"=w440) -> ("Output"=w433:dbl)
        n239 = property on="Z-axis control" class="Slide (strict)"("Value"=w434) -> ()  [unwired: 2 in, 2 out]
        n240 = property on="X-axis control" class="Slide (strict)"("Value"=w435) -> ()  [unwired: 2 in, 2 out]
        n241 = property on="Theta-angle control" class="Slide (strict)"("Value"=w433) -> ()  [unwired: 2 in, 2 out]
      }
      frame #3 {
        # "PI-controller"
        n242 = Subtract(x=w471, y=w469) -> (x-y=w470:dbl)
        n243 = Subtract(x=w465, y=w466) -> (x-y=w461:dbl)
        n244 = Subtract(x=w468, y=w467) -> (x-y=w455:dbl)
        n245 = mathscript code="act_PID = 0;\n\nif abs(d_theta) > 0.1\nact_PID = 0; % P controller\nend\n\nif abs(d_theta)>0.005 && abs(d_theta)<=0.1\nact_PID = 1; % PI controller\nend\n\nif abs(d_theta) <= 0.005\nact_PID = 2; % Stop controller\nend"("d_theta"=w461) -> ("act_PID"=w456:i32)  [unwired: 1 in, 1 out]
        n246 = mathscript code="act_PID = 0;\n\nif abs(d_x) > 0.2\nact_PID = 0; % P controller\nend\n\nif abs(d_x)>0.03 && abs(d_x)<=0.2\nact_PID = 1; % PI controller\nend\n\nif abs(d_x) <= 0.03\nact_PID = 2; % Stop controller\nend"("d_x"=w455) -> ("act_PID"=w450:i32)  [unwired: 1 in, 1 out]
        n247 = call "deadzone.vi"("threshold"=0.05, "in"=w470) -> ("out"=w472:dbl)
        n248 = case shown="0, Default" w456 {
          tunnel: w461 -> [w564 w569 _]
          tunnel: [w563 w572 0.0] -> w460
          tunnel: [0 w568 0.0] -> w458
          tunnel: [0 0 0] -> w457
          frame #0 {
            n249 = Multiply(x=w564, y=4.0) -> (x*y=w563:dbl)
          }
          frame #1 {
            n250 = feedback #4() -> (w571:dbl)  [unwired: 1 in]
            n251 = Add(x=w569, y=w571) -> (x+y=w570:dbl)
            n252 = Multiply(x=w570, y=0.04) -> (x*y=w568:dbl)
            n253 = Multiply(x=w569, y=4.0) -> (x*y=w572:dbl)
          }
          frame #2 {
          }
        }
        n254 = case shown="1" w450 {
          tunnel: w455 -> [w483 w488 _]
          tunnel: [w482 w491 0.0] -> w453
          tunnel: [0 w487 0.0] -> w452
          tunnel: [0 0 0] -> w451
          frame #0 {
            n255 = Multiply(x=w483, y=0.4) -> (x*y=w482:dbl)
          }
          frame #1 {
            n256 = feedback #5() -> (w490:dbl)  [unwired: 1 in]
            n257 = Add(x=w488, y=w490) -> (x+y=w489:dbl)
            n258 = Multiply(x=w488, y=0.05) -> (x*y=w491:dbl)
            n259 = Multiply(x=w489, y=0.005) -> (x*y=w487:dbl)
          }
          frame #2 {
          }
        }
        n260 = Multiply(x=w472, y=0.5) -> (x*y=w475:dbl)
        n261 = call "Saturation.vi"("Limit"=1.0, "Input"=w475) -> ("Output"=w464:dbl)
        n262 = property on="Z-axis control" class="Slide (strict)"("Value"=w464) -> ()  [unwired: 2 in, 2 out]
        n263 = Compound Arithmetic op=ADD(w460, w458, w457) -> (w459:dbl)
        n264 = Compound Arithmetic op=ADD(w453, w452, w451) -> (w454:dbl)
        n265 = call "Saturation.vi"("Limit"=1.0, "Input"=w459) -> ("Output"=w462:dbl)
        n266 = call "Saturation.vi"("Limit"=1.0, "Input"=w454) -> ("Output"=w463:dbl)
        n267 = property on="Theta-angle control" class="Slide (strict)"("Value"=w462) -> ()  [unwired: 2 in, 2 out]
        n268 = property on="X-axis control" class="Slide (strict)"("Value"=w463) -> ()  [unwired: 2 in, 2 out]
      }
      frame #4 {
        # "PID-controller, with oscillation dampening"
        n269 = call "Delay_region_sample_control_v3.vi"("K2"=w650, "K1"=w651, "Z"=w652, "X"=w653, "Beta"=w654, "Alpha"=w655) -> ("delta_T"=w647:dbl, "delta_X"=w648:dbl, "delta_Z"=w649:dbl)  [unwired: 1 in]
        n270 = call "Saturation.vi"("Limit"=1.0) -> ("Output"=w664:dbl)  [unwired: 1 in]
        n271 = property on="Theta-angle control" class="Slide (strict)"("Value"=w664) -> ()  [unwired: 2 in, 2 out]
        n272 = Add(x=w681, y=w649) -> (x+y=w678:dbl)
        n273 = Add(x=w680, y=w648) -> (x+y=w677:dbl)
        n274 = Add(x=w679, y=w647) -> (x+y=w676:dbl)
        n275 = Subtract(x=w678, y=w652) -> (x-y=w667:dbl)
        n276 = Subtract(x=w677, y=w653) -> (x-y=w645:dbl)
        n277 = Subtract(x=w676, y=w675) -> (x-y=w656:dbl)
        n278 = mathscript code="act_PID = 0;\n\nif abs(d_x) > 0.1\nact_PID = 0; % P controller\nend\n\nif abs(d_x)>0.05 && abs(d_x)<=0.1\nact_PID = 1; % PID controller\nend\n\nif abs(d_x) <= 0.05\nact_PID = 2; % Stop controller\nend"("d_x"=w645) -> ("act_PID"=w646:i32)  [unwired: 1 in, 1 out]
        n279 = mathscript code="act_PID = 0;\n\nif abs(d_theta) > 0.1\nact_PID = 0; % P controller\nend\n\nif abs(d_theta)>0.01 && abs(d_theta)<=0.1\nact_PID = 1; % PID controller\nend\n\nif abs(d_theta) <= 0.01\nact_PID = 2; % Stop controller\nend"("d_theta"=w656) -> ("act_PID"=w657:i32)  [unwired: 1 in, 1 out]
        n280 = call "deadzone.vi"("threshold"=0.08, "in"=w667) -> ("out"=w668:dbl)
        n281 = case shown="1" w646 {
          tunnel: w645 -> [w686 w695 _]
          tunnel: [w685 w699 0.0] -> w643
          tunnel: [0 w696 0.0] -> w642
          tunnel: [0 w692 0] -> w641
          frame #0 {
            n282 = Multiply(x=w686, y=0.4) -> (x*y=w685:dbl)
          }
          frame #1 {
            n283 = local read "Z displacement chart"() -> (w688:dbl)
            n284 = local read "Z displacement chart"() -> (w689:dbl)
            n285 = feedback #6() -> (w698:dbl)  [unwired: 1 in]
            n286 = Add(x=w695, y=w698) -> (x+y=w697:dbl)
            n287 = feedback #7() -> (w694:dbl)  [unwired: 1 in]
            n288 = mathscript code="Kp = -0.000625*z + 0.35;"("z"=w688) -> ("Kp"=w691:dbl)  [unwired: 1 in, 1 out]
            n289 = mathscript code="Kd = -0.0063*z + 2;"("z"=w689) -> ("Kd"=w687:dbl)  [unwired: 1 in, 1 out]
            n290 = Multiply(x=w697, y=0.004) -> (x*y=w696:dbl)
            n291 = Subtract(x=w695, y=w694) -> (x-y=w693:dbl)
            n292 = Multiply(x=w695, y=w691) -> (x*y=w699:dbl)
            n293 = Multiply(x=w693, y=w687) -> (x*y=w692:dbl)
          }
          frame #2 {
          }
        }
        n294 = case shown="1" w657 {
          tunnel: w656 -> [w812 w820 _]
          tunnel: [w811 w824 0.0] -> w661
          tunnel: [0 w821 0.0] -> w659
          tunnel: [0 w817 0] -> w658
          frame #0 {
            n295 = Multiply(x=w812, y=4.0) -> (x*y=w811:dbl)
          }
          frame #1 {
            n296 = feedback #8() -> (w819:dbl)  [unwired: 1 in]
            n297 = local read "Z displacement chart"() -> (w816:dbl)
            n298 = Subtract(x=w820, y=w819) -> (x-y=w818:dbl)
            n299 = feedback #9() -> (w823:dbl)  [unwired: 1 in]
            n300 = Add(x=w820, y=w823) -> (x+y=w822:dbl)
            n301 = mathscript code="Kd = 0.357*z + 20;"("z"=w816) -> ("Kd"=w815:dbl)  [unwired: 1 in, 1 out]
            n302 = Multiply(x=w822, y=0.04) -> (x*y=w821:dbl)
            n303 = Multiply(x=w818, y=w815) -> (x*y=w817:dbl)
            n304 = Multiply(x=w820, y=4.0) -> (x*y=w824:dbl)
          }
          frame #2 {
          }
        }
        n305 = Multiply(x=w668, y=0.5) -> (x*y=w672:dbl)
        n306 = call "Saturation.vi"("Limit"=1.0, "Input"=w672) -> ("Output"=w669:dbl)
        n307 = property on="Z-axis control" class="Slide (strict)"("Value"=w669) -> ()  [unwired: 2 in, 2 out]
        n308 = Compound Arithmetic op=ADD(w643, w642, w641) -> (w644:dbl)
        n309 = Compound Arithmetic op=ADD(w661, w659, w658) -> (w660:dbl)
        n310 = call "Saturation.vi"("Limit"=1.0, "Input"=w644) -> ("Output"=w670:dbl)
        n311 = call "Saturation.vi"("Limit"=1.0, "Input"=w660) -> ("Output"=w662:dbl)
        n312 = property on="X-axis control" class="Slide (strict)"("Value"=w670) -> ()  [unwired: 2 in, 2 out]
        n313 = property on="Theta-angle control" class="Slide (strict)"("Value"=w662) -> ()  [unwired: 2 in, 2 out]
      }
    }
    n314 = case shown="True" "Reset angles" {
      tunnel: w136 -> [_ w915]
      tunnel: w135 -> [_ w914]
      frame #0 {
      }
      frame #1 {
        n315 = local write "Offset Alpha"(w915) -> ()
        n316 = local write "Offset Beta"(w914) -> ()
      }
    }
    n317 = Multiply(x=w57, y=0.00582) -> (x*y=w60:dbl)
    n318 = Multiply(x=w186, y=0.00157) -> (x*y=→"Y displacement chart":dbl)
    n319 = Multiply(x=w182, y=0.00995) -> (x*y=→"Z displacement chart":dbl)
    n320 = Subtract(x=w136, y="Offset Alpha") -> (x-y=w63:dbl)
    "Encoder Alfa" <- w63
    n321 = Subtract(x=w135, y="Offset Beta") -> (x-y=w64:dbl)
    "Encoder Beta" <- w64
    n322 = To Double Precision Float(number=w225) -> (double precision float=w233:dbl)
    n323 = And(x="Saving", y=w151) -> (x .and. y?=w153:bool)
    n324 = And(x=w110, y=w109) -> (x .and. y?=w111:bool)
    n325 = Greater?(x=w200, y=1) -> (0:→"X-axis therm flag":bool)
    n326 = Greater?(x=w201, y=1) -> (0:→"T-angle therm flag":bool)
    n327 = Greater?(x=w202, y=1) -> (0:→"Z-axis therm flag":bool)
    n328 = Less?(x=w176, y=1) -> (x < y?=→"X-axis limit flag":bool)
    n329 = Less?(x=w174, y=1) -> (x < y?=→"T-angle limit flag":bool)
    n330 = Less?(x=w175, y=1) -> (x < y?=→"Z-axis limit flag":bool)
    n331 = local read "Z-axis control"() -> (w85:dbl)
    n332 = Multiply(x=w63, y=w65) -> (x*y=→"Alpha":dbl)
    n333 = Multiply(x=w64, y=w65) -> (x*y=→"Beta":dbl)
    n334 = case shown="True" w111 {
      frame #0 {
      }
      frame #1 {
        n335 = local write "Timer active"(FALSE ("Timer active")) -> ()
        n336 = property on="Load TIV" class="Bool"("DisabledEnum"=0) -> ()  [unwired: 2 in, 2 out]
        n337 = property on="Timed Sequence" class="Bool"("DisabledEnum"=0) -> ()  [unwired: 2 in, 2 out]
        n338 = property on="Stop TIV" class="Bool"("DisabledEnum"=2) -> ()  [unwired: 2 in, 2 out]
        n339 = property on="Load TIV 2" class="Path"("DisabledEnum"=T8."Enabled" ("Disabled")) -> ()  [unwired: 2 in, 2 out]
        "TIV active" <- FALSE ("TIV active")
      }
    }
    n340 = case shown="True" "Wireless Active" {
      tunnel: w60 -> [w247 _]
      tunnel: [w247 w250] -> w59
      tunnel: [w246 -1 ("pEncoder0")] -> w58
      tunnel: w57 -> [w246 _]
      frame #0 {
      }
      frame #1 {
        n341 = local read "Encoder Beta"() -> (w248:dbl)
        n342 = Divide(x=w248, y=79.14) -> (x/y=w250:dbl)
      }
    }
    "Encoder X" <- w58
    "X displacement chart" <- w59
    n343 = local read "Z displacement chart"() -> (w93:dbl)
    n344 = dll-call lib="C:/Documents and Settings/student/Desktop/crane controller/RTDACUSB_TCrane.dll" fn="RTDACUSB_Send" ("PlxApi.dll:PlxBusIopWrite")("PWMDivider"=10, "PWMWidth0"=w154, "PWMWidth1"=w166, "PWMWidth2"=w164, "PWMDir0"=w155, "PWMDir1"=w167, "PWMDir2"=w165, "PWMBrake0"=w156, "PWMBrake1"=w168, "PWMBrake2"=w68, "PWMThermFlag0"="Therm flags", "PWMThermFlag1"="Therm flags", "PWMThermFlag2"="Therm flags", "LimitFlag0"="Limit flags", "LimitFlag1"="Limit flags", "LimitFlag2"="Limit flags", "Limit0"=133, "Limit1"=29, "Limit2"=156, "EncoderReset0"=w189, "EncoderReset1"=w189, "EncoderReset2"=w189, "EncoderReset3"=w189, "EncoderReset4"=w189, "EncoderAutoResetFlag0"=w219, "EncoderAutoResetFlag1"=w219, "EncoderAutoResetFlag2"=w219, "TmrCnt0_Reset"=0, "TmrCnt0_Mode"=1) -> ()  [unwired: 33 in, 2 out]
    n345 = call "Convert to Dynamic Data"("Array"=w192) -> ("Dynamic Data Type"=w193:dynamicdata)  [unwired: 3 in]
    n346 = call "Convert to Dynamic Data2"("Array"=w191) -> ("Dynamic Data Type"=w195:dynamicdata)  [unwired: 3 in]
    n347 = while {
      shift-right: [w995] -> w232
      shift-left: _ -> [w994]
      tunnel: w233 -> [w995]
      tunnel: [w994] -> w231
      tunnel: FALSE -> [w993]
      stop <- w993 continue-if-true
    }
    n348 = Multiply(x=w85, y=20) -> (x*y=w83:dbl)
    n349 = call "Build XY Graph"("Y Input"=w195, "X Input"=w193) -> ("XY Graph"=→"XY Graph":cluster{"Y":dbl[], "Y":dbl[]}[])  [unwired: 8 in, 1 out]
    n350 = Merge Signals(w93, w76, w83) -> (→"Z Scope":dynamicdata)
    n351 = Subtract(x=w232, y=w231) -> (x-y=w230:dbl)
    n352 = Divide(x=w230, y=40000) -> (x/y=w227:dbl)
    "Sample time [ms]" <- w227
    n353 = local read "X-axis control"() -> (w91:dbl)
    n354 = local read "X displacement chart"() -> (w97:dbl)
    n355 = case shown="True" w153 {
      tunnel: w49 -> [_ w968]
      frame #0 {
      }
      frame #1 {
        w964 = FALSE
        n356 = property on="Start saving" class="Bool"("DisabledEnum"=0) -> ()  [unwired: 2 in, 2 out]
        n357 = local write "Saving"(w964) -> ()
        n358 = property on="Stop saving" class="Bool"("DisabledEnum"=2) -> ()  [unwired: 2 in, 2 out]
        n359 = local write "Timer active"(w964) -> ()
        n360 = Build Array("];", "t = cdm(:,1);\nx=cdm(:,2);\ntheta = cdm(:,3);\nz = cdm(:,4);\nalpha =cdm(:,5);\nbeta = cdm(:,6);\nu_x = cdm(:,7);\nu_theta = cdm(:,8);\nu_z = cdm(:,9);\nTs = cdm(:,10);\n") -> (w967:string[])
        n361 = call-poly <vilib>:"Write To Spreadsheet File.vi"("delimiter (\\t)"="\r\n", "append to file? (new file:F)"=TRUE, "1D data"=w967, "file path (dialog if empty)"=w968) -> ()  [unwired: 4 in, 1 out]
      }
    }
    n362 = stacked-sequence {
      tunnel: w49 -> [_ _ w376]
      frame #0 {
        # "Update the timer"
        n363 = case shown="True" "Timer active" {
          frame #0 {
          }
          frame #1 {
            n364 = local read "Sample time [ms]"() -> (w344:dbl)
            n365 = Add(x=107374.182375 ("y"), y=w344) -> (x+y=w343:dbl)
            n366 = Less Than 0?(x=w344) -> (x < 0?=w342:bool)
            n367 = Select(t=w343, s=w342, f=w344) -> (s? t:f=w341:dbl)
            n368 = Divide(x=w341, y=1000.0) -> (x/y=w339:dbl)
            n369 = local read "Time"() -> (w338:dbl)
            n370 = Add(x=w339, y=w338) -> (x+y=w346:dbl)
            n371 = local write "Time"(w346) -> ()
          }
        }
      }
      frame #1 {
        n372 = local read "TIV active"() -> (w347:bool)
        n373 = case shown="True" w347 {
          frame #0 {
          }
          frame #1 {
            # "If it's time to switch, load new values"
            n374 = local read "Switch at"() -> (w349:dbl)
            n375 = local read "Time"() -> (w350:dbl)
            n376 = Greater Or Equal?(x=w350, y=w349) -> (x >= y?=w348:bool)
            n377 = case shown="True" w348 {
              frame #0 {
              }
              frame #1 {
                n378 = stacked-sequence {
                  frame #0 {
                    n379 = local read "Index"() -> (w356:i32)
                    n380 = local read "TIV Table"() -> (w353:string[][])
                    n381 = Increment(x=w356) -> (x+1=w363:i32)
                    n382 = Decrement(x=w356) -> (x-1=w354:i32)
                    n383 = local read "Input type"() -> (w361:bool)
                    n384 = call "TIV extract element.vi"("Column"=0, "Row"=w363, "Table"=w353) -> ("Element"=→"Switch at":dbl)
                    n385 = call "TIV extract element.vi"("Column"=2, "Row"=w356, "Table"=w353) -> ("Element"=w359:dbl)
                    n386 = call "TIV extract element.vi"("Column"=1, "Row"=w356, "Table"=w353) -> ("Element"=w358:dbl)
                    n387 = call "TIV extract element.vi"("Column"=3, "Row"=w356, "Table"=w353) -> ("Element"=w360:dbl)
                    n388 = call "TIV extract element.vi"("Column"=1, "Row"=w354, "Table"=w353) -> ("Element"=w351:dbl)
                    n389 = call "TIV extract element.vi"("Column"=2, "Row"=w354, "Table"=w353) -> ("Element"=w352:dbl)
                    n390 = case shown="True" w361 {
                      tunnel: w360 -> [w369 w371]
                      tunnel: w359 -> [w370 w372]
                      tunnel: w358 -> [w368 w373]
                      tunnel: w352 -> [_ _]
                      tunnel: w351 -> [_ _]
                      frame #0 {
                        # "Set loaded values as control signals"
                        n391 = property on="Theta-angle control" class="Slide (strict)"("Value"=w370) -> ()  [unwired: 2 in, 2 out]
                        n392 = property on="X-axis control" class="Slide (strict)"("Value"=w368) -> ()  [unwired: 2 in, 2 out]
                        n393 = property on="Z-axis control" class="Slide (strict)"("Value"=w369) -> ()  [unwired: 2 in, 2 out]
                      }
                      frame #1 {
                        # "Set loaded values as reference signals"
                        n394 = property on="T" class="DigNum (strict)"("Value"=w372) -> ()  [unwired: 2 in, 2 out]
                        n395 = property on="Z" class="DigNum (strict)"("Value"=w371) -> ()  [unwired: 2 in, 2 out]
                        n396 = property on="X" class="DigNum (strict)"("Value"=w373) -> ()  [unwired: 2 in, 2 out]
                      }
                    }
                  }
                  frame #1 {
                    n397 = local read "Index"() -> (w375:i32)
                    n398 = Increment(x=w375) -> (x+1=→"Index":i32)
                  }
                }
              }
            }
          }
        }
      }
      frame #2 {
        n399 = local read "Saving"() -> (w377:bool)
        n400 = case shown="True" w377 {
          tunnel: w376 -> [_ w390]
          frame #0 {
          }
          frame #1 {
            # "Write data to file"
            n401 = local read "Y displacement chart"() -> (w387:dbl)
            n402 = local read "Z displacement chart"() -> (w386:dbl)
            n403 = local read "X displacement chart"() -> (w388:dbl)
            n404 = local read "Sample time [ms]"() -> (w381:dbl)
            n405 = local read "Numeric 2"() -> (w383:dbl)
            n406 = local read "Numeric 3"() -> (w382:dbl)
            n407 = local read "Numeric"() -> (w384:dbl)
            n408 = local read "Alpha"() -> (w379:dbl)
            n409 = local read "Beta"() -> (w378:dbl)
            n410 = local read "Time"() -> (w380:dbl)
            n411 = Build Array(w380, w388, w387, w386, w379, w378, w384, w383, w382, w381) -> (w389:dbl[])
            n412 = call-poly <vilib>:"Write To Spreadsheet File.vi"("format (%.3f)"="%.;%.4f", "append to file? (new file:F)"=TRUE, "1D data"=w389, "file path (dialog if empty)"=w390) -> ()  [unwired: 4 in, 1 out]
          }
        }
      }
    }
    n413 = To Long Integer(number=w227) -> (32bit integer=→"Waveform Chart":i32)
    n414 = Multiply(x=w91, y=40) -> (x*y=w89:dbl)
    n415 = Merge Signals(w97, w80, w89) -> (→"X Scope":dynamicdata)
    n416 = node-c288() -> ()  [unwired: 1 in, 1 out]
    "X - Motor On/Off" <- "X-Motor On/Off"
    "Numeric" <- "X-axis control"
    "Theta - Motor On/Off" <- "T-Motor On/Off"
    "Numeric 2" <- "Theta-angle control"
    "Z - Motor On/Off" <- "Z-Motor On/Off"
    "Numeric 3" <- "Z-axis control"
    "Reference Series\n(Trajectory)" <- "Input type"
  }
  n417 = node-c288(w20) -> ()  [unwired: 1 out]
  n418 = VISA Close(VISA resource name=w3, error in (no error)=w2) -> (error out=w4:errorcluster)
  n419 = call <vilib>:"Simple Error Handler.vi"("error in (no error)"=w4) -> ()  [unwired: 1 in, 8 out]
